vi "Update Calibration (Date).vi"(5 "New Calibration Password":string, 6 "Remote Timeout (300,000 ms)":u32=300000, 7 "Calibration Password":string, 8 "error in (no error)":errorcluster, 9 "Calibration Due Date":timestamp, 10 "Calibration Date":timestamp, 11 "Resource in":refnum<k20>) -> (0 "error out":errorcluster, 2 "Detailed Result":string, 3 "Resource out":refnum<k20>)   [LabVIEW 2014, in "nisyscfg.lvlib"]
doc: "Updates the external calibration information for a device. You can only use this VI to update calibration information if the Supports Calibration Write property is TRUE."
uses:
  nisyscfg.lvlib
  C:/Program Files (x86)/National Instruments/LabVIEW 2014/resource/objmgr/nisysapi.rc
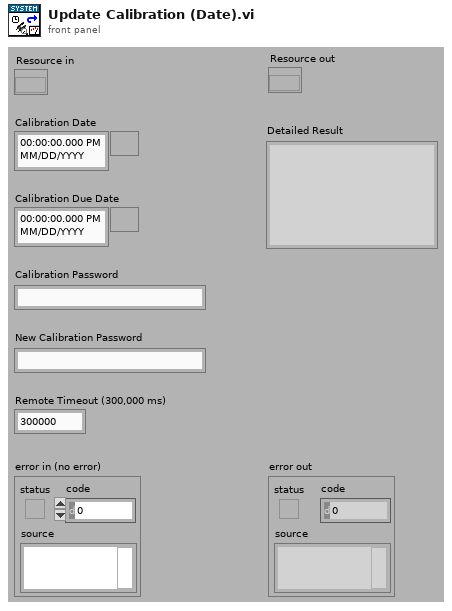
[diagram p1: front panel]
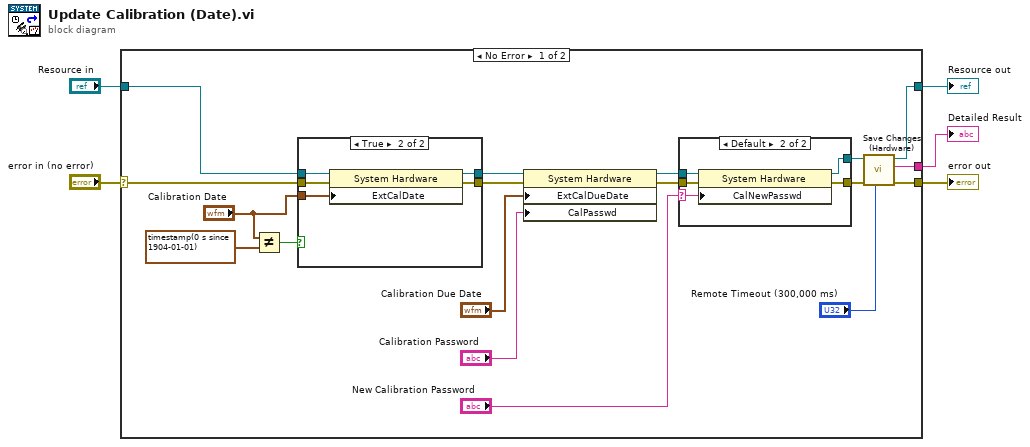
[diagram p0: block diagram]
diagram:
  n1 = case shown="No Error" "error in (no error)" {
    selector: "error in (no error)" -> [w21 w39]
    tunnel: [w11 w39] -> w5
    tunnel: "Resource in" -> [w22 w38]
    tunnel: [w10 _] -> w2
    tunnel: [w9 w38] -> w1
    frame No Error {
      n2 = Not Equal?(x="Calibration Date", y=timestamp(0 s since 1904-01-01) ("Time")) -> (x != y?=w23:bool)
      n3 = case shown="True" w23 {
        tunnel: w22 -> [w32 w37]
        tunnel: w21 -> [w31 w36]
        tunnel: "Calibration Date" -> [_ w35]
        tunnel: [w32 w34] -> w20
        tunnel: [w31 w33] -> w19
        frame False {
        }
        frame True {
          n4 = property class="System Hardware"(reference=w37, error in=w36, "ExtCalDate"=w35) -> (reference out=w34:refnum<k20>, error out=w33:errorcluster)
        }
      }
      n5 = property class="System Hardware"(reference=w20, error in=w19, "ExtCalDueDate"="Calibration Due Date", "CalPasswd"="Calibration Password") -> (reference out=w15:refnum<k20>, error out=w16:errorcluster)
      n6 = case shown="Default" "New Calibration Password" {
        selector: "New Calibration Password" -> [_ w28]
        tunnel: w16 -> [w24 w30]
        tunnel: w15 -> [w25 w29]
        tunnel: [w24 w27] -> w12
        tunnel: [w25 w26] -> w13
        frame "" {
        }
        frame Default {
          n7 = property class="System Hardware"(reference=w29, error in=w30, "CalNewPasswd"=w28) -> (reference out=w26:refnum<k20>, error out=w27:errorcluster)
        }
      }
      n8 = call "Save Changes (Hardware).vi"("Remote Timeout (300,000 ms)"="Remote Timeout (300,000 ms)", "error in (no error)"=w12, "Resource in"=w13) -> ("error out"=w11:errorcluster, "Detailed Result"=w10:string, "Resource out"=w9:refnum<k20>)  [unwired: 5 in, 1 out]
    }
    frame Error {
    }
  }
  "error out" <- w5
  "Resource out" <- w1
  "Detailed Result" <- w2
